vi "CMD_SERIALPRINT.vi"(6 "Gantry in":refnum<class "Gantry.lvclass">, 7 "Console Log in":refnum<class "Console Log.lvclass">, 8 "error in (no error)":errorcluster, 10 "Arguments":string[](array[string]), 11 "gScript Interpreter in":refnum<class "gScript Interpreter.lvclass">) -> (0 "error out":errorcluster, 3 "gScript Interpreter out":refnum<class "gScript Interpreter.lvclass">, 4 "Gantry out":refnum<class "Gantry.lvclass">, 5 "Console Log out":refnum<class "Console Log.lvclass">)   [LabVIEW 2023, in "gScript Interpreter.lvclass"]
uses:
  gScript Interpreter.lvclass
  Shared Components/Gantry Class/Gantry.lvclass
  Application Utilities/Console Log/Console Log.lvclass
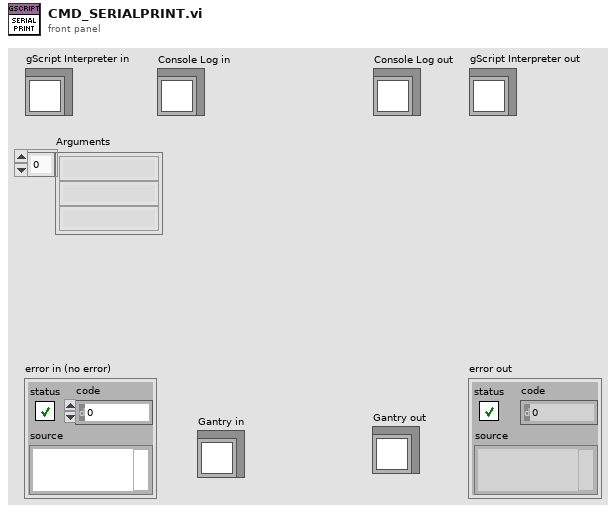
[diagram p1: front panel]
types:
  T1 = typedef "Memory Cell.ctl" = cluster{"type":T2, "x":dbl, "y":dbl, "z":dbl, "w":dbl}
  T2 = typedef "Memory Cell Type Enum.ctl" = enum16{"integer", "float", "vector", "rotation"}
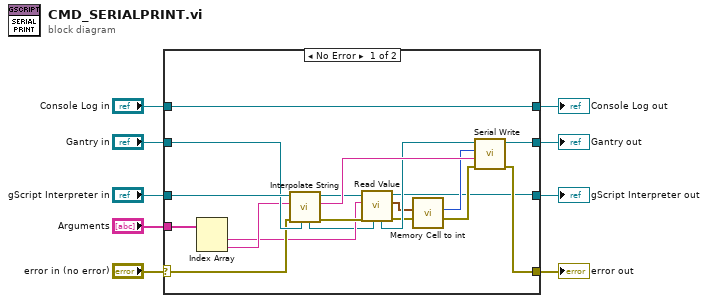
[diagram p0: block diagram]
diagram:
  n1 = case shown="No Error" "error in (no error)" {
    selector: "error in (no error)" -> [w22 w31]
    tunnel: [w11 w31] -> w8
    tunnel: [w10 w30] -> w6
    tunnel: "gScript Interpreter in" -> [w26 w30]
    tunnel: "Arguments" -> [w24 _]
    tunnel: "Gantry in" -> [w25 w29]
    tunnel: [w12 w29] -> w3
    tunnel: "Console Log in" -> [w27 w28]
    tunnel: [w27 w28] -> w1
    frame No Error {
      n2 = Index Array(array=w24) -> (element #1=w18:string, element #2=w23:string)  [unwired: 2 in]
      n3 = call-dynamic "Interpolate String.vi"("Gantry in"=w25, "error in (no error)"=w22, "Input String"=w23, "gScript Interpreter in"=w26) -> ("error out"=w20:errorcluster, "Output String"=w21:string, "gScript Interpreter out"=w19:refnum<class "gScript Interpreter.lvclass">, "Gantry out"=w17:refnum<class "Gantry.lvclass">)  [unwired: 4 in]
      n4 = call-dynamic "Read Value.vi"("Gantry in"=w17, "error in (no error)"=w20, "String in"=w18, "gScript Interpreter in"=w19) -> ("error out"=w14:errorcluster, "Memory Cell"=w15:T1, "gScript Interpreter out"=w10:refnum<class "gScript Interpreter.lvclass">, "Gantry out"=w16:refnum<class "Gantry.lvclass">)  [unwired: 4 in]
      n5 = call "Memory Cell to int.vi"("Memory Cell"=w15) -> ("Int out"=w13:i32)  [unwired: 10 in]
      n6 = call "Serial Write.vi"("error in (no error)"=w14, "Write Buffer"=w21, "Connection ID"=w13, "Gantry in"=w16) -> ("error out"=w11:errorcluster, "Gantry out"=w12:refnum<class "Gantry.lvclass">)  [unwired: 5 in, 1 out]
    }
    frame Error {
    }
  }
  "error out" <- w8
  "gScript Interpreter out" <- w6
  "Gantry out" <- w3
  "Console Log out" <- w1
